vi "Remove call chain from error message.vi"(1 "Error message in":string) -> (0 "Error message out (text before call chain)":string)   [LabVIEW 2020, in "status_text_indicator.lvlib"]
uses:
  Status_Text_Indicator.lvlib
panel:
  # "Development\ncontrols/indicators useful for development and testing, but which are not outputs of the VI"
  # "Input\nInputs to the VI"
  # "Output\nOutputs of the VI"
  # "Description\n\nBlank VI with error handling case. \n\nSummarize the use of this VI in this space."
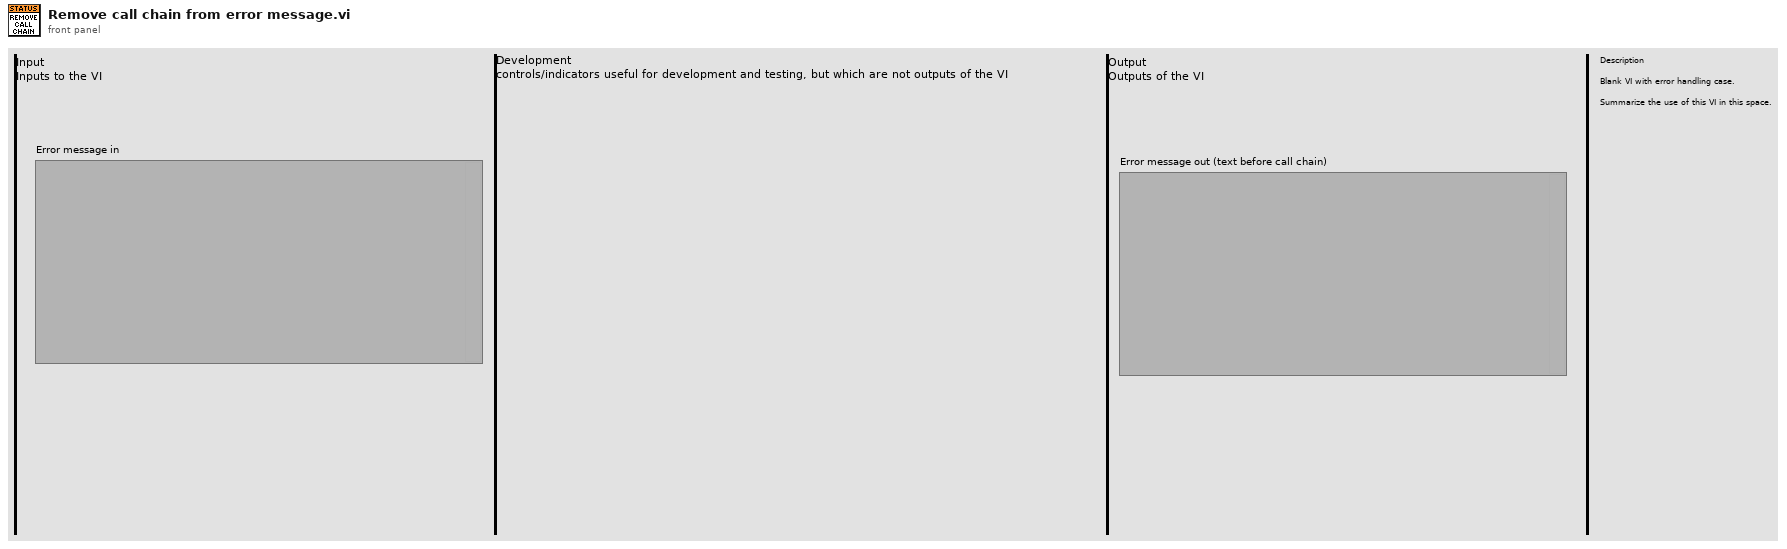
[diagram p1: front panel]
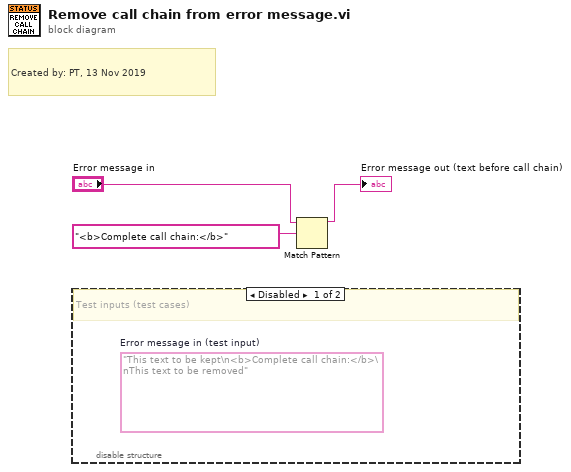
[diagram p0: block diagram]
diagram:
  # "Created by: PT, 13 Nov 2019"
  n1 = disable-structure shown="Disabled" {
    frame Disabled {
      (unwired) "This text to be kept\n<b>Complete call chain:</b>\nThis text to be removed"  # Error message in (test input)
      # "Test inputs (test cases)"
    }
    frame Enabled {
    }
  }
  n2 = Match Pattern(string="Error message in", regular expression="<b>Complete call chain:</b>") -> (before substring=→"Error message out (text before call chain)":string)  [unwired: 1 in, 3 out]
